vi "currently listening.vi"(11 "Queue server in":refnum<class "Queue server.lvclass">) -> (3 "listening?":bool)   [LabVIEW 2015, in "Queue server.lvclass"]
uses:
  Queue server.lvclass
  Queue server.lvclass/Queue server.ctl
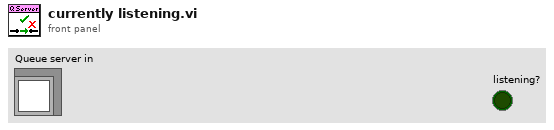
[diagram p1: front panel]
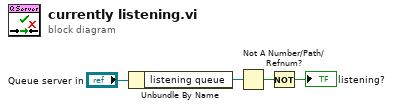
[diagram p0: block diagram]
diagram:
  n1 = Unbundle By Name("Queue server in") -> ("listening queue"=w3:refnum<queue>)
  n2 = Not A Number/Path/Refnum?(number/path/refnum=w3) -> (NaN/Path/Refnum?=w2:bool)
  n3 = Not(x=w2) -> (.not. x?=→"listening?":bool)
